vi "Append Image To Document.vi"() -> ()   [LabVIEW 2017]
doc: "Demonstrates how to add an image to an MS Office document."
uses:
  LabVIEW NPOI/Document/Document.lvclass
panel:
  out "XY Graph":cluster{dbl[], dbl[]}(graph)={[0.0, 0.19866933079506122, 0.3894183423086505, 0.5646424733950355, 0.7173560908995228, 0.8414709848078965, 0.9320390859672264, 0.9854497299884603, 0.9995736030415051, 0.9738476308781951, 0.9092974268256817, 0.8084964038195901, 0.6754631805511506, 0.5155013718214642, 0.33498815015590466, 0.1411200080598672, -0.058374143427580086, -0.25554110202683167, -0.44252044329485246, -0.6118578909427193, -0.7568024953079282, -0.8715757724135882, -0.951602073889516, -0.9936910036334645, -0.9961646088358406, -0.9589242746631385, -0.8834546557201531, -0.7727644875559871, -0.6312666378723208, -0.4646021794137566, -0.27941549819892586, -0.0830894028174964, 0.11654920485049364, 0.3115413635133787, 0.49411335113860894, 0.6569865987187891, 0.7936678638491531, 0.8987080958116269, 0.9679196720314865, 0.998543345374605, 0.9893582466233818, 0.9407305566797726, 0.8545989080882804, 0.7343970978741133, 0.5849171928917617, 0.4121184852417566, 0.22288991410024592, 0.024775425453357765, -0.1743267812229814, -0.36647912925192844, -0.5440211108893698, -0.6998746875935437, -0.8278264690856537, -0.9227754216128073, -0.9809362300664916, -0.9999902065507035, -0.979177729151317, -0.9193285256646757, -0.8228285949687079, -0.6935250847771224, -0.5365729180004349, -0.35822928223682704, -0.1656041754483094, 0.03362304722113847, 0.23150982510153895, 0.4201670368266409, 0.5920735147072245, 0.7403758899524486, 0.8591618148564968, 0.9436956694441048, 0.9906073556948704, 0.9980266527163616, 0.9656577765492774, 0.8947911721405034, 0.7882520673753163, 0.6502878401571168, 0.4863986888537981, 0.30311835674570226, 0.1077536522994423, -0.09190685022768164, -0.2879033166650653, -0.47242198639846616, -0.6381066823479502, -0.7783520785342984, -0.8875670335815046, -0.9613974918795568, -0.9969000660415961, -0.9926593804706327, -0.948844497918124, -0.8672021794855813, -0.750987246771676, -0.6048328224062841, -0.43456562207189353, -0.2469736617366209, -0.04953564087836742, 0.14987720966295234, 0.3433149288198987, 0.5230657651576994, 0.6819636200681356, 0.8136737375071054], [1.0, 0.955336489125606, 0.8253356149096783, 0.6216099682706645, 0.3623577544766736, 0.0707372016677029, -0.2272020946930869, -0.5048461045998576, -0.7373937155412454, -0.904072142017061, -0.9899924966004454, -0.9874797699088649, -0.8967584163341472, -0.7259323042001402, -0.4902608213406994, -0.2107957994307797, 0.0874989834394464, 0.37797774271298024, 0.6346928759426339, 0.8347127848391598, 0.960170286650366, 0.9998586363834151, 0.9502325919585296, 0.8157251001253574, 0.6083513145322552, 0.3466353178350258, 0.05395542056264975, -0.2435441537357911, -0.5192886541166856, -0.7486466455973987, -0.9111302618846769, -0.9922253254526032, -0.984687855794127, -0.8891911526253609, -0.7142656520272003, -0.4755369279959925, -0.19432990645533654, 0.10423602686569687, 0.3934908663478909, 0.6475963386538759, 0.8438539587324921, 0.9647326178866094, 0.9994345855010047, 0.9448600381598606, 0.8058839576404507, 0.594920663309892, 0.3308148779490486, 0.03715838479082641, -0.2598173562137541, -0.5335843865891177, -0.7596879128588213, -0.9179307804142925, -0.9941776251838151, -0.9816175436063848, -0.8813724903622346, -0.7023970575027135, -0.46067858741136253, -0.17780907112311914, 0.12094359992847414, 0.4088927393988798, 0.6603167082440802, 0.8527565521308732, 0.969022192939049, 0.9987279672435017, 0.9392203466968708, 0.7958149698139441, 0.5813218118144357, 0.3149009076879376, 0.02035084333168298, -0.27601710124946705, -0.5477292602242684, -0.7705143956585688, -0.9244717749141202, -0.9958488438257794, -0.9782697014065075, -0.8733046400935156, -0.6903298762015725, -0.4456900004443363, -0.16123796432418885, 0.1376169789418758, 0.424179007336997, 0.6728503883183468, 0.861418048028701, 0.9730377990279994, 0.9977389813911304, 0.933315112063922, 0.7855209834229068, 0.5675586048115467, 0.2988979063644716, 0.003537548134909945, -0.2921388087338362, -0.5617192758811498, -0.7811230330551121, -0.9307513960668837, -0.9972385088794737, -0.9746452757206577, -0.8649898828201904, -0.6780675198445613, -0.43057540477663, -0.1446212711617233]}
  out "File Path":path
  in  "Document Format":enum16{"xlsx", "xls", "docx", "doc"}(ring)
  # "Overview: Demonstrates how to add an image to an MS Office document.\nInstructions:\n1. Entre a Document Name and select the Document Format you want to create.\n2. Run the VI.\n3. The generated document will be located at the path indicated by File Path.\n4. Delete the temporary Document file when you are done."
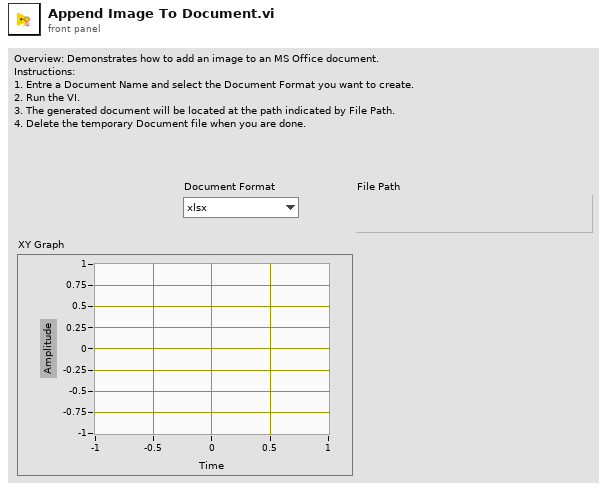
[diagram p1: front panel]
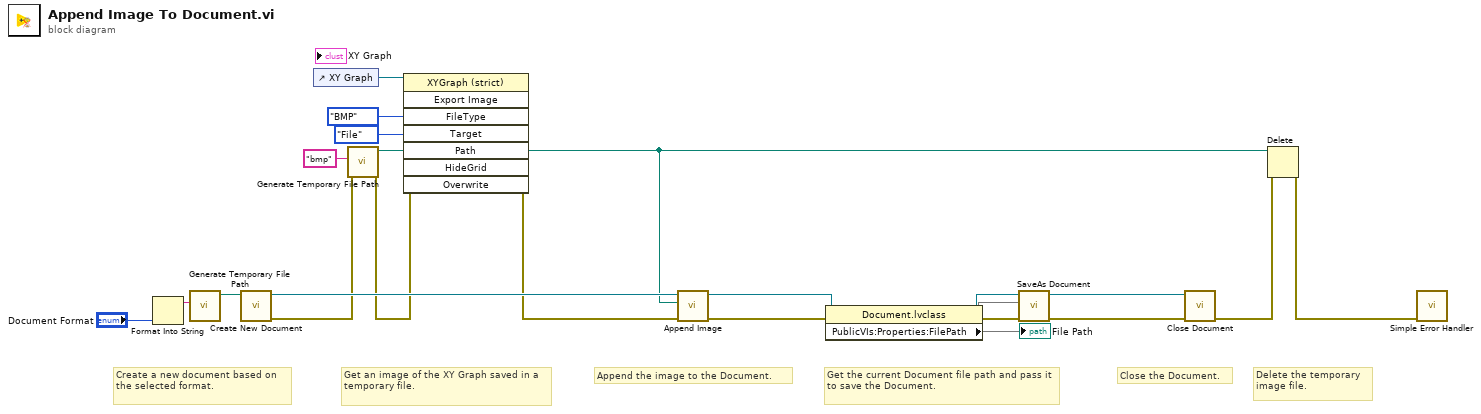
[diagram p0: block diagram]
diagram:
  # "Create a new document based on the selected format."
  # "Delete the temporary image file."
  # "Close the Document."
  # "Get the current Document file path and pass it to save the Document."
  # "Append the image to the Document."
  # "Get an image of the XY Graph saved in a temporary file."
  n1 = Format Into String("Document Format") -> (resulting string=w3:string)  [unwired: 3 in, 1 out]
  n2 = call <vilib>:"Generate Temporary File Path.vi"("Temporary File Extension (tmp)"=w3) -> ("Unique Temporary File Path"=w2:path)  [unwired: 9 in, 1 out]
  n3 = call "Create New Document.vi"("File Path"=w2) -> ("error out"=w7:errorcluster, "Document out"=w21:refnum<class "Document.lvclass">)  [unwired: 9 in]
  n4 = control-ref of="XY Graph"() -> (w4:refnum<vi>)
  n5 = call <vilib>:"Generate Temporary File Path.vi"("error in (no error)"=w7, "Temporary File Extension (tmp)"="bmp") -> ("error out"=w6:errorcluster, "Unique Temporary File Path"=w17:path)  [unwired: 8 in]
  n6 = invoke on="Invoke Node" class="XYGraph (strict)" method="Export Image"(reference=w4, error in=w6, "FileType"=enum32{"BMP", "EPS", "EMF", "PICT"}."BMP" ("File Type"), "Target"=enum32{"File", "Clipboard"}."File", "Path"=w17) -> (error out=w5:errorcluster)  [unwired: 3 in, 7 out]
  n7 = call "Append Image.vi"("error in (no error)"=w5, "Image File Path"=w17, "Document in"=w21) -> ("error out"=w11:errorcluster, "Document out"=w12:refnum<class "Document.lvclass">)  [unwired: 7 in]
  n8 = property class="Document.lvclass"(reference=w12, error in=w11) -> (reference out=w14:refnum<class "Document.lvclass">, error out=w16:errorcluster, "PublicVIs:Properties:FilePath"=w13)
  "File Path" <- w13
  n9 = call "SaveAs Document.vi"("error in (no error)"=w16, "File Path"=w13, "Document in"=w14) -> ("error out"=w15:errorcluster, "Document out"=w10:refnum<class "Document.lvclass">)  [unwired: 7 in]
  n10 = call "Close Document.vi"("error in (no error)"=w15, "Document in"=w10) -> ("error out"=w9:errorcluster)  [unwired: 9 in]
  n11 = Delete(path (use dialog)=w17, error in=w9) -> (error out=w8:errorcluster)  [unwired: 3 in, 2 out]
  n12 = call <vilib>:"Simple Error Handler.vi"("error in (no error)"=w8) -> ()  [unwired: 4 in, 5 out]
